vi "Add to queue.vi"(8 "error in (no error)":errorcluster, 9 "timeout in ms (-1)":i32=-1, 10 "Data":variant, 11 "Message in":refnum<class "Message.lvclass">) -> (0 "error out":errorcluster, 3 "Message out":refnum<class "Message.lvclass">)   [LabVIEW 2015, in "Message.lvclass"]
uses:
  Message.lvclass
  Message.lvclass/Message.ctl
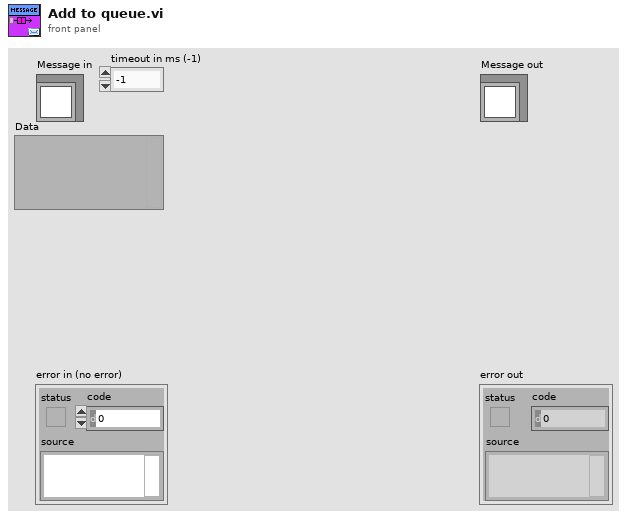
[diagram p1: front panel]
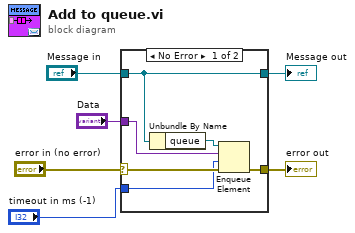
[diagram p0: block diagram]
diagram:
  n1 = case shown="No Error" "error in (no error)" {
    selector: "error in (no error)" -> [w10 w14]
    tunnel: [w9 w14] -> w5
    tunnel: [w8 w13] -> w3
    tunnel: "Message in" -> [w8 w13]
    tunnel: "Data" -> [w11 _]
    tunnel: "timeout in ms (-1)" -> [w7 _]
    frame No Error {
      n2 = Unbundle By Name(w8) -> ("queue"=w12:refnum<queue>)
      n3 = Enqueue Element(queue=w12, element=w11, timeout in ms (-1)=w7, error in (no error)=w10) -> (error out=w9:errorcluster)  [unwired: 2 out]
    }
    frame Error {
    }
  }
  "error out" <- w5
  "Message out" <- w3
